vi "SaveTemplate.vi"() -> ()   [LabVIEW 2016]
uses:
  VIs/ColorText/Code.xctl
panel:
  in  "VISA resource name":refnum<visa-resource-name>
  in  "Open":bool
  in  "Save Button":bool
  in  "Code":string(xcontrol)
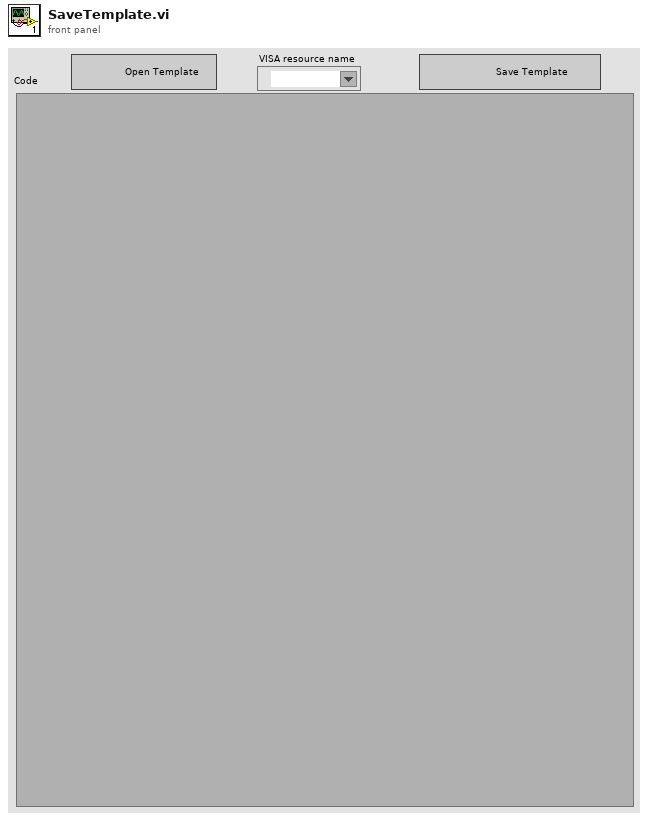
[diagram p1: front panel]
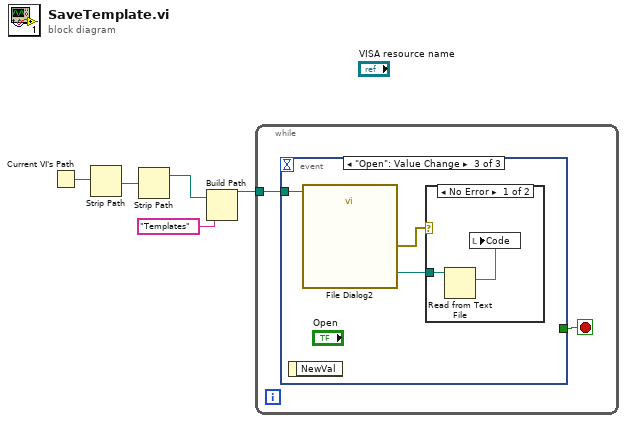
[diagram p0: block diagram]
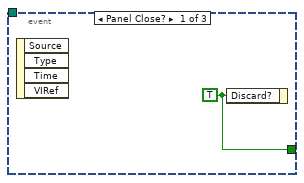
[diagram p2: hidden frame]
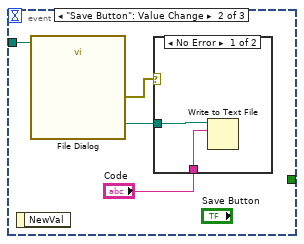
[diagram p3: hidden frame]
diagram:
  n1 = Current VI's Path() -> (path=w4:path)
  n2 = Strip Path(path=w4) -> (stripped path=w3:path)  [unwired: 1 out]
  n3 = Strip Path(path=w3) -> (stripped path=w2:path)  [unwired: 1 out]
  n4 = Build Path(base path=w2, name or relative path="Templates") -> (appended path=w1:path)
  n5 = while {
    tunnel: w1 -> [w6]
    stop <- w7 stop-if-true
    n6 = event shown="[2] \"Open\": Value Change" {
      selector: _ -> [_ _ _]
      dyn-events: _ -> [_ _ _]
      timeout: _ -> [_ _ _]
      tunnel: [w8 _ _] -> w7
      tunnel: w6 -> [_ w10 w16]
      event Panel Close? {
        w8 = TRUE ("Discard?")
        n7 = event-data() -> ()  [unwired: 1 in, 4 out]
        n8 = event-data("Discard?"=w8) -> ()  [unwired: 1 in, 1 out]
      }
      event "Save Button": Value Change {
        n9 = event-data() -> ()  [unwired: 1 in, 1 out]
        n10 = call "File Dialog"("start path"=w10) -> ("selected path"=w12:path, "error out"=w9:errorcluster)  [unwired: 11 in, 2 out]
        n11 = case shown="No Error" w9 {
          tunnel: w12 -> [w14 _]
          tunnel: "Code" -> [w13 _]
          frame No Error {
            n12 = Write to Text File(file (use dialog)=w14, text=w13) -> ()  [unwired: 2 in, 3 out]
          }
          frame Error {
          }
        }
      }
      event "Open": Value Change {
        n13 = event-data() -> ()  [unwired: 1 in, 1 out]
        n14 = call "File Dialog2"("start path"=w16) -> ("selected path"=w17:path, "error out"=w15:errorcluster)  [unwired: 11 in, 2 out]
        n15 = case shown="No Error" w15 {
          tunnel: w17 -> [w19 _]
          frame No Error {
            n16 = Read from Text File(file (use dialog)=w19) -> (text=w18:string)  [unwired: 3 in, 3 out]
            n17 = local write "Code"(w18) -> ()
          }
          frame Error {
          }
        }
      }
    }
  }
